vi "Generate_2D_Raster.vi"(8 "error in (no error)":errorcluster, 10 "Y Parameters":T2, 11 "X Parameters":T1) -> (0 "error IO":errorcluster, 3 "Array":dbl[][](array[numeric]))   [LabVIEW 2012]
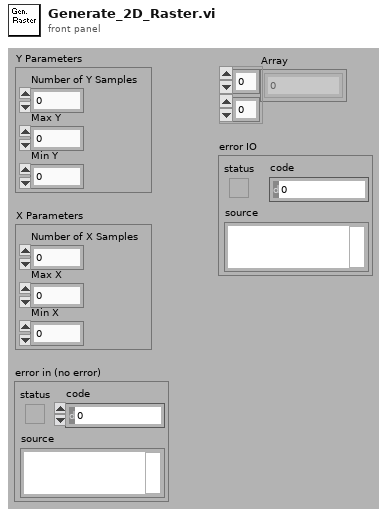
[diagram p1: front panel]
types:
  T1 = cluster{"Number of X Samples":i32, "Max X":dbl, "Min X":dbl}
  T2 = cluster{"Number of Y Samples":i32, "Max Y":dbl, "Min Y":dbl}
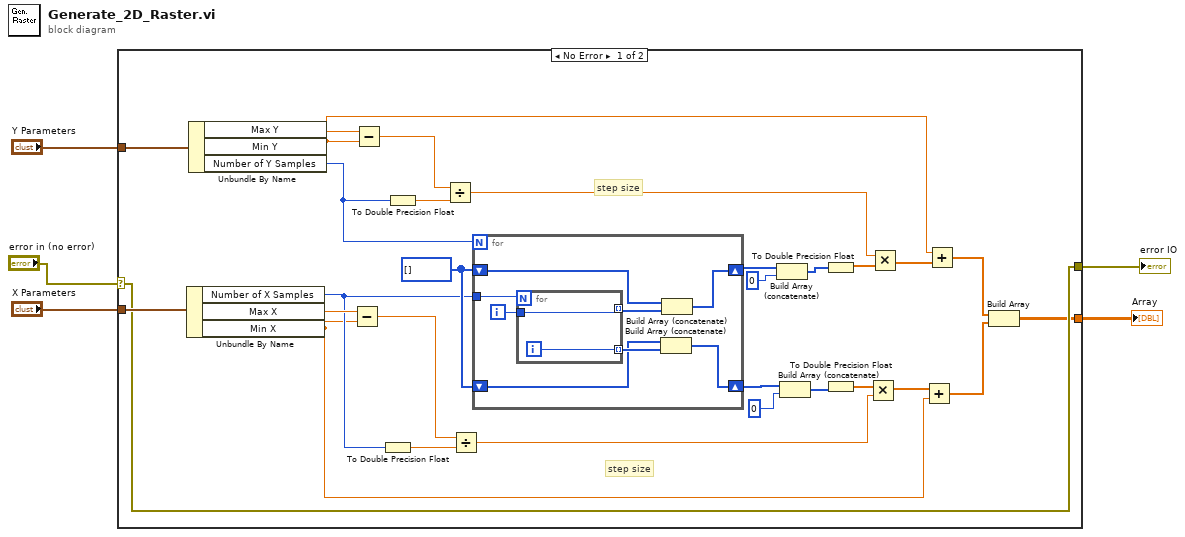
[diagram p0: block diagram]
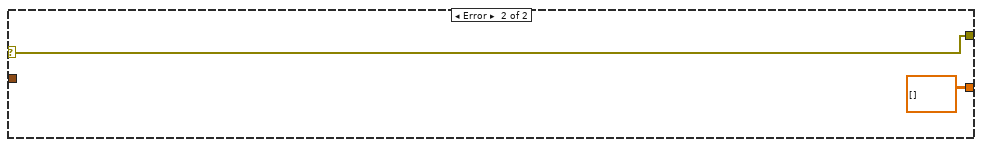
[diagram p2: hidden frame]
diagram:
  n1 = case shown="No Error" "error in (no error)" {
    selector: "error in (no error)" -> [w13 w46]
    tunnel: "X Parameters" -> [w34 _]
    tunnel: "Y Parameters" -> [w33 _]
    tunnel: [w6 dbl[][] []] -> w3
    tunnel: [w13 w46] -> w5
    frame No Error {
      w23 = i32[] []
      # "step size"
      # "step size"
      n2 = Unbundle By Name(w34) -> ("Number of X Samples"=w20:i32, "Max X"=w31:dbl, "Min X"=w17:dbl)
      n3 = Unbundle By Name(w33) -> ("Max Y"=w32:dbl, "Min Y"=w24:dbl, "Number of Y Samples"=w29:i32)
      n4 = Subtract(x=w31, y=w17) -> (x-y=w22:dbl)
      n5 = Subtract(x=w32, y=w24) -> (x-y=w30:dbl)
      n6 = To Double Precision Float(number=w20) -> (double precision float=w21:dbl)
      n7 = To Double Precision Float(number=w29) -> (double precision float=w28:dbl)
      n8 = Divide(x=w30, y=w28) -> (x/y=w26:dbl)
      n9 = Divide(x=w22, y=w21) -> (x/y=w18:dbl)
      n10 = for {
        N: w29 -> [_]
        shift-right: [w38] -> w10
        shift-left: w23 -> [w36]
        shift-right: [w39] -> w12
        shift-left: w23 -> [w37]
        tunnel: w20 -> [w35]
        i -> [w42]
        n11 = for {
          N: w35 -> [_]
          tunnel: [w44] -> w40 mode=indexing
          tunnel: w42 -> [w44]
          tunnel: [w43] -> w41 mode=indexing
          i -> [w43]
        }
        n12 = Build Array (concatenate)(w36, w41) -> (w38:i32[])
        n13 = Build Array (concatenate)(w37, w40) -> (w39:i32[])
      }
      n14 = Build Array (concatenate)(w12, 0) -> (w9:i32[])
      n15 = Build Array (concatenate)(w10, 0) -> (w8:i32[])
      n16 = To Double Precision Float(number=w9) -> (double precision float=w27:dbl[])
      n17 = To Double Precision Float(number=w8) -> (double precision float=w19:dbl[])
      n18 = Multiply(x=w19, y=w18) -> (x*y=w16:dbl[])
      n19 = Multiply(x=w26, y=w27) -> (x*y=w25:dbl[])
      n20 = Add(x=w16, y=w17) -> (x+y=w14:dbl[])
      n21 = Add(x=w24, y=w25) -> (x+y=w15:dbl[])
      n22 = Build Array(w15, w14) -> (w6:dbl[][])
    }
    frame Error {
    }
  }
  "error IO" <- w5
  "Array" <- w3
